vi "DSB_SC(SubVI).vi"(4 "message amplitude":dbl(slide)=1.0 scale=0.0..1.0, 5 "modulation frequency":dbl(knob)=10.0 scale=0.0..1000.0, 6 "sampling info":cluster{"Fs":dbl, "#s":dbl}, 7 "carrier frequency":dbl(knob)=10.0 scale=0.0..500000.0) -> (0 "baseband signal (time-domain)":waveform(dbl)(graph), 1 "baseband signal (frequency-domain)":cluster{"f0":dbl, "df":dbl, "magnitude":dbl[]}(graph), 2 "Baseband/AM":dbl, 3 "modulated signal (time-domain)":waveform(dbl)(graph))   [LabVIEW 2010]
uses:
  <vilib>/measure/maspectr.llb/FFT Spectrum (Mag-Phase) for 1 Chan.vi
  <vilib>/measure/NI_MABase.lvlib
  <vilib>/measure/NI_MAPro.lvlib
  <vilib>/ptbypt/NI_PtbyPt.lvlib
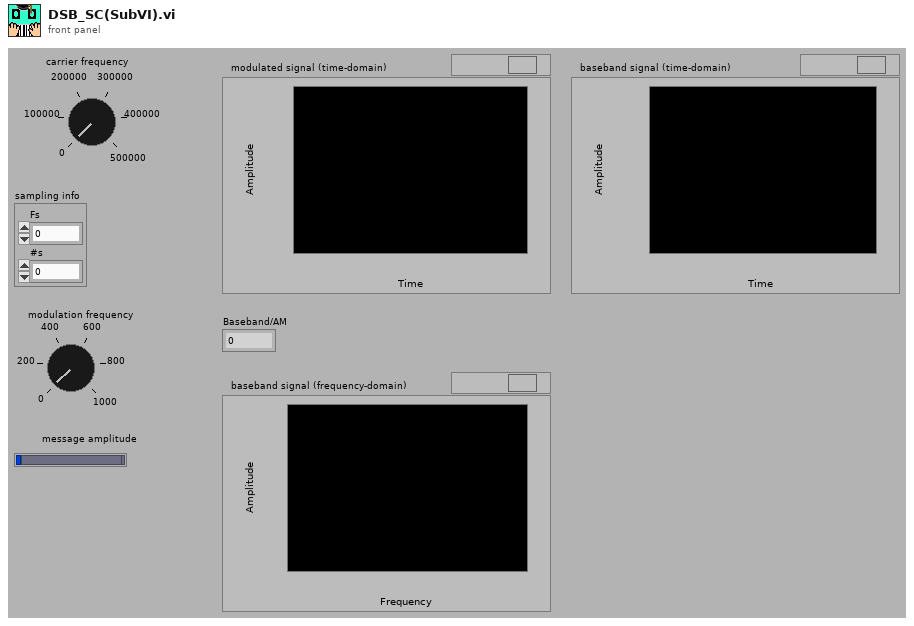
[diagram p1: front panel]
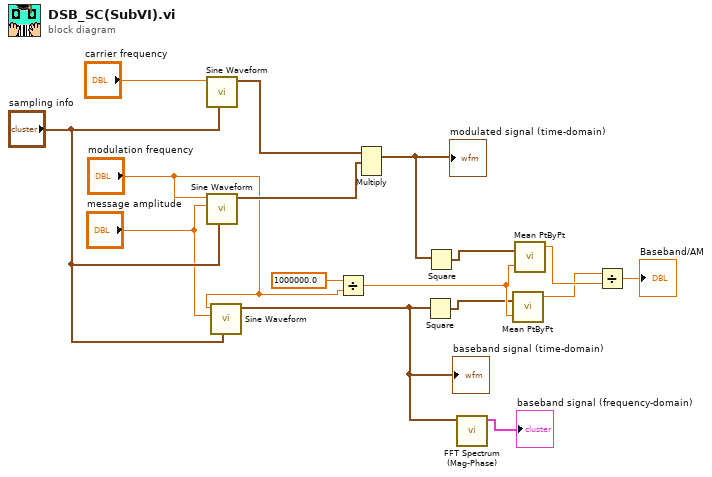
[diagram p0: block diagram]
diagram:
  n1 = call <vilib>:"Sine Waveform.vi"("sampling info"="sampling info", "frequency"="carrier frequency") -> ("signal out"=w3:waveform(dbl))  [unwired: 8 in, 1 out]
  n2 = call <vilib>:"Sine Waveform.vi"("sampling info"="sampling info", "amplitude"="message amplitude", "frequency"="modulation frequency") -> ("signal out"=w16:waveform(dbl))  [unwired: 7 in, 1 out]
  n3 = call <vilib>:"Sine Waveform.vi"("sampling info"="sampling info", "amplitude"="message amplitude", "frequency"="modulation frequency") -> ("signal out"=w13:waveform(dbl))  [unwired: 7 in, 1 out]
  "baseband signal (time-domain)" <- w13
  n4 = Divide(x=1000000.0, y="modulation frequency") -> (x/y=w9:dbl)
  n5 = Multiply(1:w16, 2:w3) -> (0:w5:waveform(dbl))  [unwired: 1 in, 1 out]
  "modulated signal (time-domain)" <- w5
  n6 = Square(x=w13) -> (x^2=w6:waveform(dbl))
  n7 = Square(x=w5) -> (x^2=w7:waveform(dbl))
  n8 = call-poly <vilib>:"FFT Spectrum (Mag-Phase).vi"("time signal"=w13) -> ("magnitude"=→"baseband signal (frequency-domain)":cluster{"f0":dbl, "df":dbl, "magnitude":dbl[]})  [unwired: 6 in, 4 out]
  n9 = call <vilib>:"Mean PtByPt.vi"("x"=w6, "sample length"=w9) -> ("mean"=w11:dbl)  [unwired: 2 in, 1 out]
  n10 = call <vilib>:"Mean PtByPt.vi"("x"=w7, "sample length"=w9) -> ("mean"=w12:dbl)  [unwired: 2 in, 1 out]
  n11 = Divide(x=w11, y=w12) -> (x/y=→"Baseband/AM":dbl)
